vi "Gyroscope Event Example.vi"() -> ()   [LabVIEW 2012, in "Phidget Gyroscope.lvlib"]
uses:
  <instrlib>/Phidgets/Phidget Gyroscope/Phidget Gyroscope.lvlib
  <instrlib>/Phidgets/Phidget Gyroscope/Public/GyroscopeStart.vi
  <instrlib>/Phidgets/Phidget Gyroscope/Public/GyroscopeClose.vi
  <instrlib>/Phidgets/Phidget Common/Phidget Common.lvlib
panel:
  out "Timestamp":u64
  in  "stop":bool
  out "Serial Number Return":i32
  in  "Device Info":T1={"Serial Number"=-1, "Channel"=0, "Port"=0}
  out "Angular Rate Data":dbl[](array[numeric])
  out "error out":errorcluster
  # "Be sure to use this stop button to stop the program.\nIf you use the \"Abort Execution\" button, you will\nneed to use PhidgetResetLibrary.vi or restart Labview \nin order for any Phidgets to work."
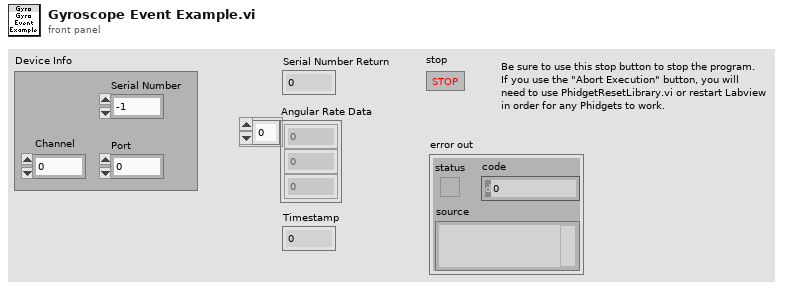
[diagram p1: front panel]
types:
  T1 = cluster{"Serial Number":i32, "Channel":i32, "Port":i32}
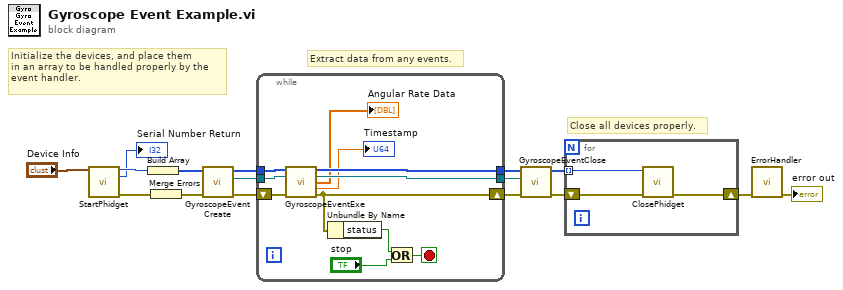
[diagram p0: block diagram]
diagram:
  # "Close all devices properly."
  # "Extract data from any events."
  # "Initialize the devices, and place them\nin an array to be handled properly by the\nevent handler."
  n1 = call-poly <instrlib>:"StartPhidget.vi"("Device Info"="Device Info") -> ("Phidget ID"=w5:u64, "Serial Number Return"=→"Serial Number Return":i32, "error out"=w2:errorcluster)  [unwired: 11 in, 1 out]
  n2 = Build Array(w5) -> (w16:u64[])
  n3 = Merge Errors(w2) -> (w7:errorcluster)
  n4 = call <instrlib>:"GyroscopeEventCreate.vi"("error in (no error)"=w7, "Devices In"=w16) -> ("error out"=w9:errorcluster, "Event Registration Refnum"=w14:refnum<event-registration>, "Devices Out"=w15:u64[])  [unwired: 7 in]
  n5 = while {
    tunnel: w15 -> [w27]
    tunnel: w14 -> [w23]
    tunnel: [w26] -> w11
    shift-right: [w22] -> w10
    shift-left: w9 -> [w25]
    tunnel: [w24] -> w3
    stop <- w21 stop-if-true
    n6 = call <instrlib>:"GyroscopeEventExe.vi"("Devices In"=w27, "Event Registration Refnum In"=w23, "error in (no error)"=w25) -> ("Devices Out"=w24:u64[], "Event Registration Refnum Out"=w26:refnum<event-registration>, "Gyro Data"=→"Angular Rate Data":dbl[], "Timestamp"=→"Timestamp":dbl, "error out"=w22:errorcluster)  [unwired: 5 in, 3 out]
    n7 = Unbundle By Name(w22) -> ("status"=w19:bool)
    n8 = Or(x=w19, y="stop") -> (x .or. y?=w21:bool)
  }
  n9 = call <instrlib>:"GyroscopeEventClose.vi"("error in (no error)"=w10, "Event Registration Refnum In"=w11, "Devices In"=w3) -> ("error out"=w6:errorcluster, "Devices Out"=w4:u64[])  [unwired: 7 in]
  n10 = for {
    tunnel: w4 -> [w28] mode=indexing
    shift-right: [w30] -> w13
    shift-left: w6 -> [w29]
    n11 = call-poly <instrlib>:"ClosePhidget.vi"("error in"=w29, "Device In"=w28) -> ("error out"=w30:errorcluster)  [unwired: 9 in]
  }
  n12 = call <instrlib>:"ErrorHandler.vi"("error in"=w13) -> ("error out"=→"error out":errorcluster)  [unwired: 9 in, 1 out]
